vi "Rotation Control.vi"(8 "error in (no error)":errorcluster, 11 "Control Panel in":refnum<class "Control Panel.lvclass">) -> (0 "error out":errorcluster, 3 "Control Panel out":refnum<class "Control Panel.lvclass">)   [LabVIEW 2019, in "Control Panel.lvlib" / "Control Panel.lvclass"]
uses:
  Control Panel.lvclass
  <vilib>/Rock Robotics/WPI/ThirdParty/Phoenix-LabVIEW/Motor Controller/Controls/CTRE_Phoenix_MotorControl_ControlMode.ctl
panel:
  out "Changes":i32
  out "Matched Color Name":string
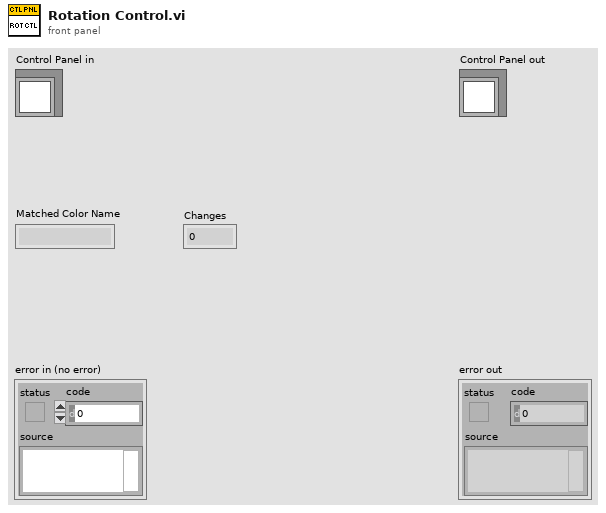
[diagram p1: front panel]
types:
  T1 = typedef "CTRE_Phoenix_MotorControl_ControlMode.ctl" = u16
  T2 = typedef "Color Sensor V3 DevRef.ctl" = cluster{"I2CDevRef":T3}
  T3 = typedef "WPI_I2CDevRef.ctl" = cluster{"DevStatus":errorcluster, "Device Address":u8, "Handle":i32, "I2C Bus":T4}
  T4 = typedef "i2c_bus.ctl" = enum16{"I2C On-Board", "I2C MXP", "Invalid"}
  T5 = typedef "WPI_MotorControlDeviceRef.ctl" = cluster{"DeviceStatus":errorcluster, "Type":T6, "PWM":cluster{"PWM Channel":T7, "DeadBand":T8}, "CAN":cluster{"Device Number":u8, "SetOutput VI Ref":variant, "GetOutput VI Ref":variant, "Enable VI Ref":variant, "Disable VI Ref":variant, "Data":variant}, "Invert":bool, "DIO PWM":cluster{"PWM \"Enable\" Channel":T7, "DIOChannel":T9, "PWM Rate":dbl}}
  T6 = typedef "WPI_MotorControlType.ctl" = enum16{"PWM", "CAN", "DIO PWM"}
  T7 = typedef "FPGA_DIOPWMChannel.ctl" = enum8{"PWM 0", "PWM 1", "PWM 2", "PWM 3", "PWM 4", "PWM 5", "PWM 6", "PWM 7", "PWM 8", "PWM 9", "PWM MXP 0", "PWM MXP 1", "PWM MXP 2", "PWM MXP 3", "PWM MXP 4", "PWM MXP 5", "PWM MXP 6", "PWM MXP 7", "PWM MXP 8", "PWM MXP 9", "Invalid"}
  T8 = typedef "WPI_PWMDeadband.ctl" = cluster{"Name":string, "maxPositivePwm":i32, "minPositivePwm":i32, "centerPwm":i32, "maxNegativePwm":i32, "minNegativePwm":i32, "angularRange":u16}
  T9 = typedef "FPGA_DIOChannel.ctl" = enum8{"DIO 0", "DIO 1", "DIO 2", "DIO 3", "DIO 4", "DIO 5", "DIO 6", "DIO 7", "DIO 8", "DIO 9", "DIO MXP 0", "DIO MXP 1", "DIO MXP 2", "DIO MXP 3", "DIO MXP 4", "DIO MXP 5", "DIO MXP 6", "DIO MXP 7", "DIO MXP 8", "DIO MXP 9", "DIO MXP 10", "DIO MXP 11", "DIO MXP 12", "DIO MXP 13", "DIO MXP 14", "DIO MXP 15", "SPI Port CS1", "SPI Port CS2", "SPI Port CS3", "SPI Port MISO", "SPI Port MOSI", "Invalid"}
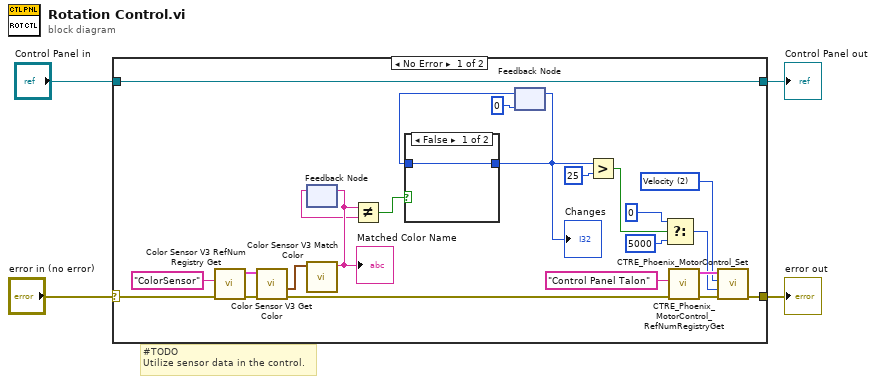
[diagram p0: block diagram]
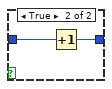
[diagram p2: hidden frame]
diagram:
  # "#TODO\nUtilize sensor data in the control."
  n1 = case shown="No Error" "error in (no error)" {
    selector: "error in (no error)" -> [w18 w32]
    tunnel: [w13 w32] -> w3
    tunnel: [w10 w31] -> w1
    tunnel: "Control Panel in" -> [w10 w31]
    frame No Error {
      w14 = T1 2 items=["PercentOutput"=0, "Position"=1, "Velocity"=2, "Current"=3, "Follower"=5, "MotionProfile"=6, "MotionMagic"=7, "MotionProfileArc"=10, "Disabled"=15] ("Control Mode")
      n2 = call <vilib>:"Color Sensor V3 RefNum Registry Get.vi"("error in (no error)"=w18, "refnum name"="ColorSensor") -> ("error out"=w22:errorcluster, "ColorSensorDevRef"=w21:T2)  [unwired: 8 in]
      n3 = call <vilib>:"Color Sensor V3 Get Color.vi"("error in (no error)"=w22, "ColorSensorDevRef"=w21) -> ("error out"=w9:errorcluster, "Normalized Color"=w23:cluster{"R":dbl, "G":dbl, "B":dbl})  [unwired: 6 in, 2 out]
      n4 = feedback #1() -> (w26:string)  [unwired: 1 in]
      n5 = call <vilib>:"Color Sensor V3 Match Color.vi"("Measured Color"=w23) -> ("Matched Color Name"=w27:string)  [unwired: 8 in, 2 out]
      "Matched Color Name" <- w27
      n6 = feedback-in #1(w27) -> ()
      n7 = Not Equal?(x=w27, y=w26) -> (x != y?=w24:bool)
      n8 = feedback #2(0) -> (w25:i32)
      n9 = case shown="False" w24 {
        tunnel: [w28 w30] -> w12
        tunnel: w25 -> [w28 w29]
        frame False {
        }
        frame True {
          n10 = Increment(x=w29) -> (x+1=w30:i32)
        }
      }
      "Changes" <- w12
      n11 = feedback-in #2(w12) -> ()
      n12 = Greater?(x=w12, y=25) -> (0:w8:bool)
      n13 = Select(t=0, s=w8, f=5000) -> (s? t:f=w5:i32)
      n14 = call <vilib>:"CTRE_Phoenix_MotorControl_RefNumRegistryGet.vi"("error in (no error)"=w9, "refnum name"="Control Panel Talon") -> ("error out"=w16:errorcluster, "PhoenixMotorControlDevRef"=w15:T5)  [unwired: 8 in]
      n15 = call <vilib>:"CTRE_Phoenix_MotorControl_Set.vi"("error in (no error)"=w16, "Output"=w5, "Control Mode"=w14, "PhoenixMotorControlDevRef"=w15) -> ("error out"=w13:errorcluster)  [unwired: 6 in, 1 out]
    }
    frame Error {
    }
  }
  "error out" <- w3
  "Control Panel out" <- w1
